vi "CalculateCheckValue.vi"(8 "error in (no error)":errorcluster, 10 "String":string, 11 "Code128 in":refnum<class "Code128.lvclass">) -> (0 "error out":errorcluster, 2 "Numeric":u8, 3 "Code128 out":refnum<class "Code128.lvclass">)   [LabVIEW 2013, in "BarCodes.lvlib" / "Code128.lvclass"]
doc: "Calculates the check value for a given input and returns it as a byte value."
uses:
  Code128.lvclass
  Code128.lvclass/Code128.ctl
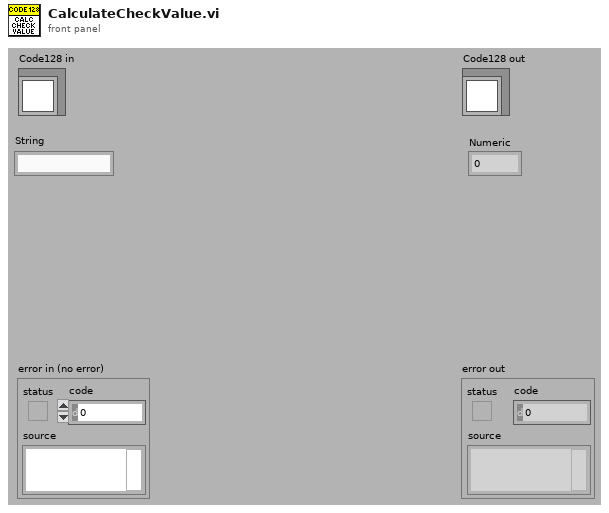
[diagram p1: front panel]
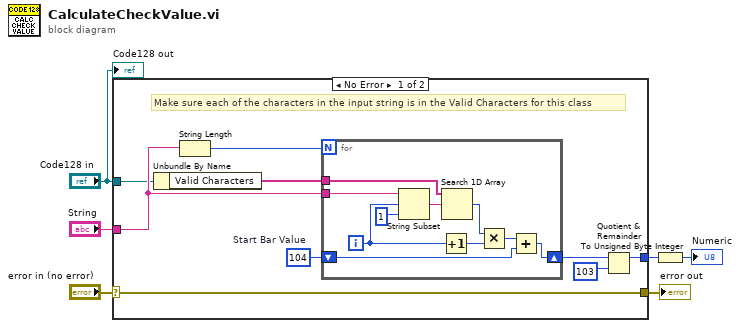
[diagram p0: block diagram]
diagram:
  n1 = case shown="No Error" "error in (no error)" {
    selector: "error in (no error)" -> [w7 w26]
    tunnel: "String" -> [w13 _]
    tunnel: [w9 _] -> w5
    tunnel: "Code128 in" -> [w8 _]
    tunnel: [w7 w26] -> w2
    frame No Error {
      w15 = 104  # Start Bar Value
      # "Make sure each of the characters in the input string is in the Valid Characters for this class"
      n2 = Unbundle By Name(w8) -> ("Valid Characters"=w12:string[])
      n3 = String Length(string=w13) -> (length=w14:i32)
      n4 = for {
        N: w14 -> [_]
        tunnel: w13 -> [w24]
        tunnel: w12 -> [w25]
        shift-right: [w16] -> w11
        shift-left: w15 -> [w17]
        i -> [w20]
        n5 = String Subset(string=w24, offset (0)=w20, length (rest)=1 ("length (rest)")) -> (substring=w21:string)
        n6 = Increment(x=w20) -> (x+1=w22:i32)
        n7 = Search 1D Array(1D array=w25, element=w21) -> (index of element=w23:i32)  [unwired: 1 in]
        n8 = Multiply(x=w23, y=w22) -> (x*y=w18:i32)
        n9 = Add(x=w18, y=w17) -> (x+y=w16:i32)
      }
      n10 = Quotient & Remainder(x=w11, y=103) -> (x-y*floor(x/y)=w9:i32)  [unwired: 1 out]
    }
    frame Error {
    }
  }
  "error out" <- w2
  n11 = To Unsigned Byte Integer(number=w5) -> (unsigned 8bit integer=→"Numeric":u8)
  "Code128 out" <- "Code128 in"
